vi "DPT CDAQ Index Array.vi"() -> (2 "CDAQ Index":string[][](array[string]), 3 "cDAQ Index":i32[][](array[numeric]))   [LabVIEW 2016]
panel:
  out "CDAQ Index Array":i32[](array[numeric])
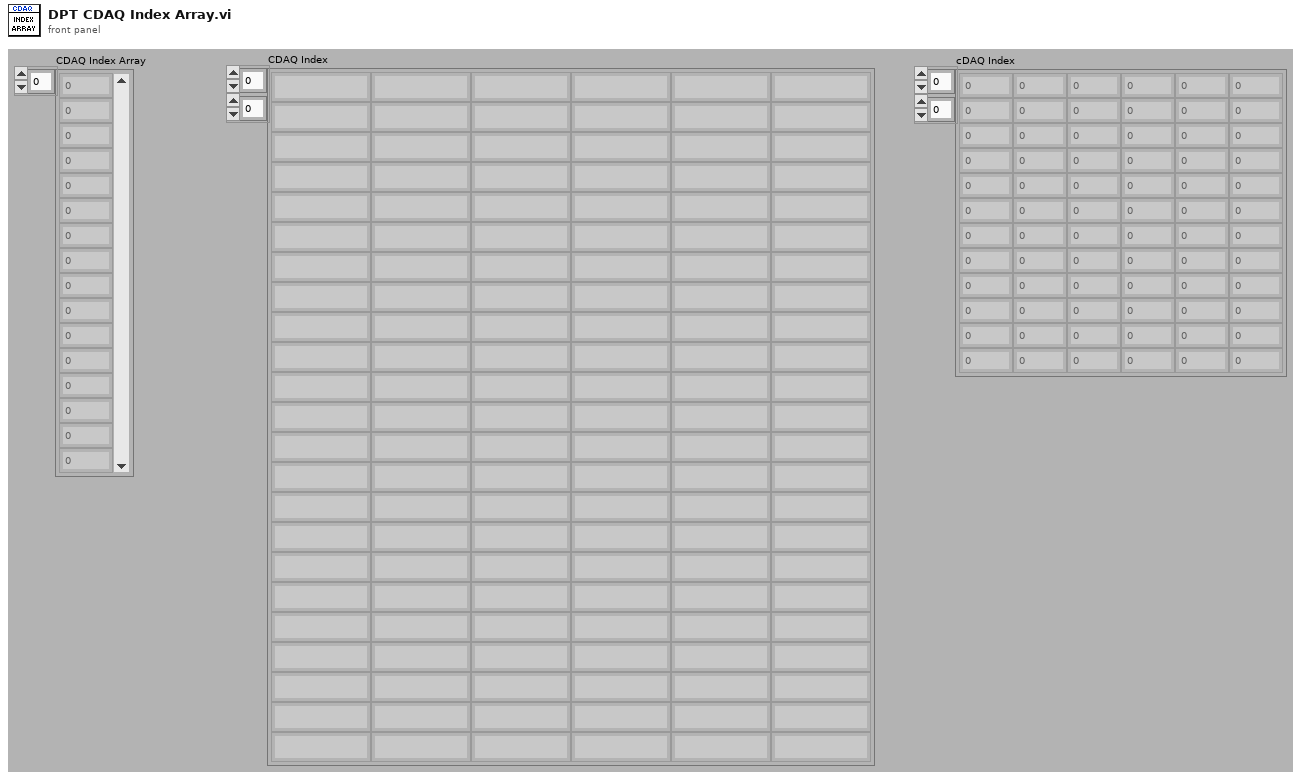
[diagram p1: front panel]
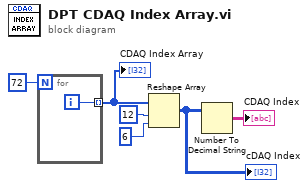
[diagram p0: block diagram]
diagram:
  n1 = for {
    N: 72 -> [_]
    tunnel: [w7] -> w6 mode=indexing
    i -> [w7]
  }
  "CDAQ Index Array" <- w6
  n2 = Reshape Array(w6, 12 ("dimension size"), 6 ("dimension size")) -> (w3:i32[][])
  "cDAQ Index" <- w3
  n3 = Number To Decimal String(number=w3) -> (decimal integer string=→"CDAQ Index":string[][])  [unwired: 1 in]
